vi "创建隐藏文件夹.vi"   [LabVIEW 2018]
uses:
  <vilib>/Utility/error.llb/DialogType.ctl
types:
  T1 = typedef "DialogType.ctl" = u16
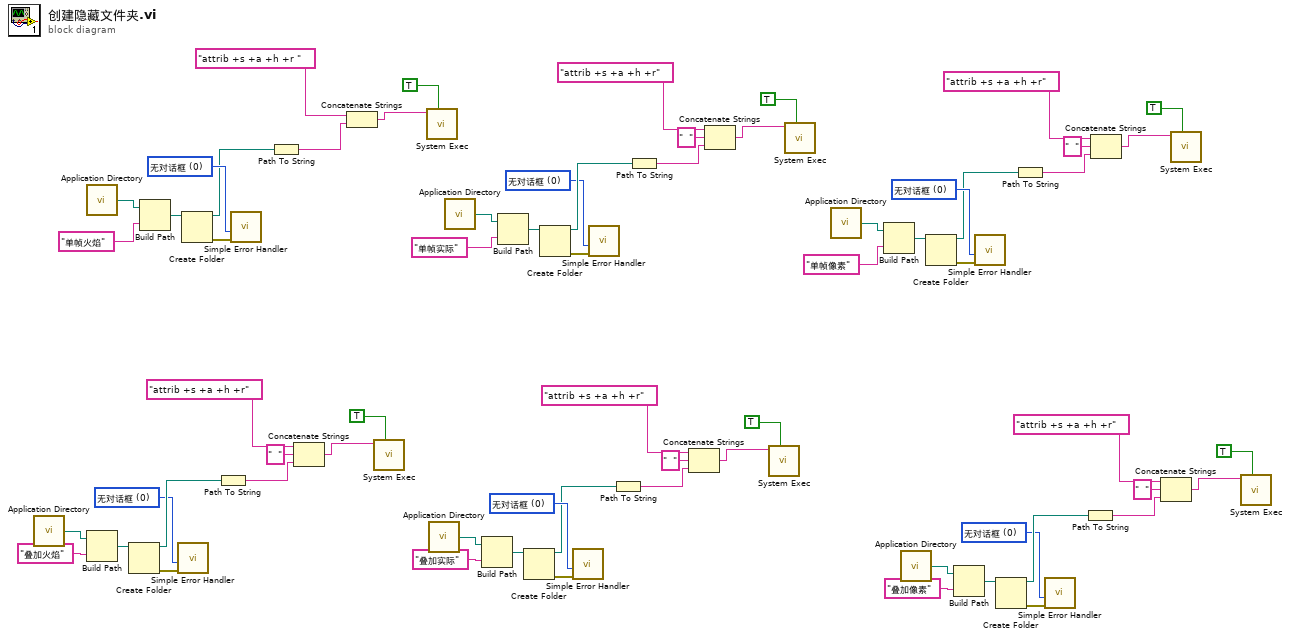
[diagram p0: block diagram]
diagram:
  w12 = T1 0 items=["无对话框", "确定信息", "继续或停止信息", "确定信息＋警告", "继续/停止+警告"] ("type of dialog (OK msg:1)")
  w23 = T1 0 items=["无对话框", "确定信息", "继续或停止信息", "确定信息＋警告", "继续/停止+警告"] ("type of dialog (OK msg:1)")
  w32 = T1 0 items=["无对话框", "确定信息", "继续或停止信息", "确定信息＋警告", "继续/停止+警告"] ("type of dialog (OK msg:1)")
  w43 = T1 0 items=["无对话框", "确定信息", "继续或停止信息", "确定信息＋警告", "继续/停止+警告"] ("type of dialog (OK msg:1)")
  w52 = T1 0 items=["无对话框", "确定信息", "继续或停止信息", "确定信息＋警告", "继续/停止+警告"] ("type of dialog (OK msg:1)")
  w61 = T1 0 items=["无对话框", "确定信息", "继续或停止信息", "确定信息＋警告", "继续/停止+警告"] ("type of dialog (OK msg:1)")
  n1 = call <vilib>:"Application Directory.vi"() -> ("Application Directory"=w28:path)
  n2 = call <vilib>:"Application Directory.vi"() -> ("Application Directory"=w65:path)
  n3 = Build Path(base path=w28, name or relative path="叠加火焰" ("名称或相对路径")) -> (appended path=w29:path)
  n4 = Create Folder(path (use dialog)=w29) -> (created path=w35:path, error out=w31:errorcluster)  [unwired: 2 in, 1 out]
  n5 = Build Path(base path=w65, name or relative path="单帧火焰" ("名称或相对路径")) -> (appended path=w64:path)
  n6 = call <vilib>:"Simple Error Handler.vi"("type of dialog (OK msg:1)"=w32, "error in (no error)"=w31) -> ()  [unwired: 3 in, 5 out]
  n7 = Create Folder(path (use dialog)=w64) -> (created path=w59:path, error out=w62:errorcluster)  [unwired: 2 in, 1 out]
  n8 = Path To String(path=w35) -> (string=w36:string)
  n9 = call <vilib>:"Simple Error Handler.vi"("type of dialog (OK msg:1)"=w61, "error in (no error)"=w62) -> ()  [unwired: 3 in, 5 out]
  n10 = Path To String(path=w59) -> (string=w7:string)
  n11 = Concatenate Strings("attrib +s +a +h +r" ("字符串"), "  " ("字符串"), w36) -> (w37:string)
  n12 = Concatenate Strings("attrib +s +a +h +r " ("字符串"), w7) -> (w58:string)
  n13 = call <vilib>:"System Exec.vi"("wait until completion? (T)"=TRUE, "command line"=w37) -> ()  [unwired: 6 in, 4 out]
  n14 = call <vilib>:"System Exec.vi"("wait until completion? (T)"=TRUE, "command line"=w58) -> ()  [unwired: 6 in, 4 out]
  n15 = call <vilib>:"Application Directory.vi"() -> ("Application Directory"=w27:path)
  n16 = call <vilib>:"Application Directory.vi"() -> ("Application Directory"=w48:path)
  n17 = Build Path(base path=w27, name or relative path="叠加实际" ("名称或相对路径")) -> (appended path=w26:path)
  n18 = Build Path(base path=w48, name or relative path="单帧实际" ("名称或相对路径")) -> (appended path=w49:path)
  n19 = Create Folder(path (use dialog)=w26) -> (created path=w20:path, error out=w24:errorcluster)  [unwired: 2 in, 1 out]
  n20 = Create Folder(path (use dialog)=w49) -> (created path=w55:path, error out=w51:errorcluster)  [unwired: 2 in, 1 out]
  n21 = call <vilib>:"Simple Error Handler.vi"("type of dialog (OK msg:1)"=w23, "error in (no error)"=w24) -> ()  [unwired: 3 in, 5 out]
  n22 = call <vilib>:"Simple Error Handler.vi"("type of dialog (OK msg:1)"=w52, "error in (no error)"=w51) -> ()  [unwired: 3 in, 5 out]
  n23 = Path To String(path=w20) -> (string=w19:string)
  n24 = Path To String(path=w55) -> (string=w56:string)
  n25 = Concatenate Strings("attrib +s +a +h +r" ("字符串"), "  " ("字符串"), w19) -> (w18:string)
  n26 = Concatenate Strings("attrib +s +a +h +r" ("字符串"), "  " ("字符串"), w56) -> (w57:string)
  n27 = call <vilib>:"System Exec.vi"("wait until completion? (T)"=TRUE, "command line"=w18) -> ()  [unwired: 6 in, 4 out]
  n28 = call <vilib>:"System Exec.vi"("wait until completion? (T)"=TRUE, "command line"=w57) -> ()  [unwired: 6 in, 4 out]
  n29 = call <vilib>:"Application Directory.vi"() -> ("Application Directory"=w47:path)
  n30 = Build Path(base path=w47, name or relative path="单帧像素" ("名称或相对路径")) -> (appended path=w46:path)
  n31 = call <vilib>:"Application Directory.vi"() -> ("Application Directory"=w8:path)
  n32 = Create Folder(path (use dialog)=w46) -> (created path=w40:path, error out=w44:errorcluster)  [unwired: 2 in, 1 out]
  n33 = Build Path(base path=w8, name or relative path="叠加像素" ("名称或相对路径")) -> (appended path=w9:path)
  n34 = call <vilib>:"Simple Error Handler.vi"("type of dialog (OK msg:1)"=w43, "error in (no error)"=w44) -> ()  [unwired: 3 in, 5 out]
  n35 = Create Folder(path (use dialog)=w9) -> (created path=w15:path, error out=w11:errorcluster)  [unwired: 2 in, 1 out]
  n36 = Path To String(path=w40) -> (string=w39:string)
  n37 = call <vilib>:"Simple Error Handler.vi"("type of dialog (OK msg:1)"=w12, "error in (no error)"=w11) -> ()  [unwired: 3 in, 5 out]
  n38 = Path To String(path=w15) -> (string=w16:string)
  n39 = Concatenate Strings("attrib +s +a +h +r" ("字符串"), "  " ("字符串"), w39) -> (w38:string)
  n40 = Concatenate Strings("attrib +s +a +h +r" ("字符串"), "  " ("字符串"), w16) -> (w17:string)
  n41 = call <vilib>:"System Exec.vi"("wait until completion? (T)"=TRUE, "command line"=w38) -> ()  [unwired: 6 in, 4 out]
  n42 = call <vilib>:"System Exec.vi"("wait until completion? (T)"=TRUE, "command line"=w17) -> ()  [unwired: 6 in, 4 out]
